vi "Reset Switch.vi"(8 "error in (no error)":errorcluster, 11 "instrument handle":refnum<k15>) -> (0 "error out":errorcluster, 3 "instrument handle out":refnum<k15>)   [LabVIEW 2015]
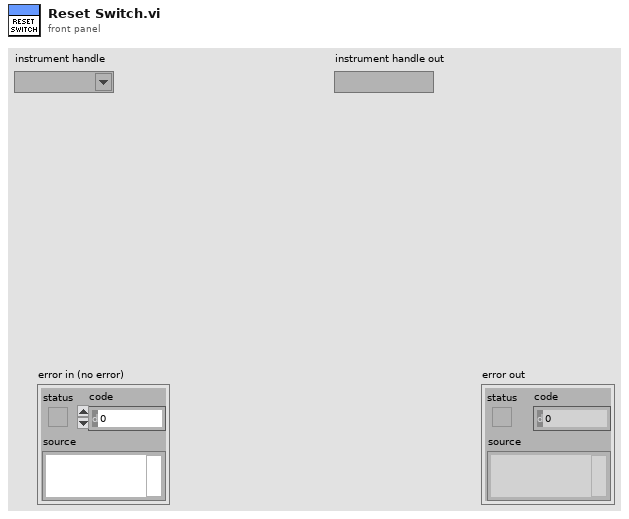
[diagram p1: front panel]
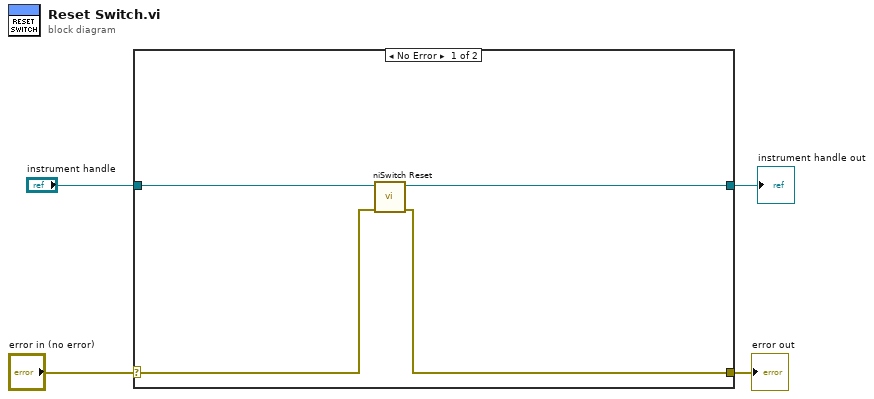
[diagram p0: block diagram]
diagram:
  n1 = case shown="No Error" "error in (no error)" {
    selector: "error in (no error)" -> [w8 w9]
    tunnel: [w7 w9] -> w3
    tunnel: "instrument handle" -> [w6 _]
    tunnel: [w5 _] -> w1
    frame No Error {
      n2 = call <instrlib>:"niSwitch Reset.vi"("error in (no error)"=w8, "instrument handle"=w6) -> ("error out"=w7:errorcluster, "instrument handle out"=w5:refnum<k15>)  [unwired: 8 in]
    }
    frame Error {
    }
  }
  "error out" <- w3
  "instrument handle out" <- w1
